vi "RunMeas.vi"(8 "error in (no error)":errorcluster, 11 "NhRegenGridSim in":refnum<class "NHRGridSim.lvclass">) -> (0 "error out":errorcluster, 2 "variant":variant, 3 "NhRegenGridSim out":refnum<class "NHRGridSim.lvclass">)   [LabVIEW 2018, in "AcPwrPlugins.lvlib" / "NHRGridSim.lvclass"]
doc: "This VI acquires data from the instrument and fetches the data from instrument memory into LabVIEW memory."
uses:
  NHRGridSim.lvclass
  AcPwrShared/clMeasurmentData.ctl
  AcPwrShared/clAcPwrAttributes.ctl
  <instrlib>/NH Research 9400 Series/Public/Data/Read Waveform (Current).vi
  <instrlib>/NH Research 9400 Series/Public/Data/Read Waveform (Voltage).vi
  <instrlib>/NH Research 9400 Series/NH Research 9400 Series.lvlib
  AcPwrShared/AcPwrShared.lvlib
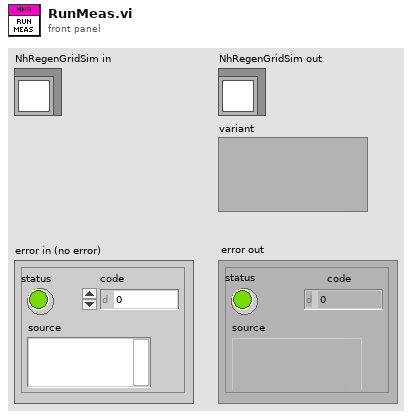
[diagram p1: front panel]
types:
  T1 = typedef "AcPwrPlugins.lvlib/NHRGridSim.lvclass/Device(s)Settings.ctl" = cluster{"MeasName":string, "Modules":T2}
  T2 = typedef "AcPwrPlugins.lvlib/NHRGridSim.lvclass/Modules.ctl" = cluster{"Measurement":cluster{"ApertureLength (s)":dbl, "NumberOfSamples":u32}, "Ranges":cluster{"Irange (A)":dbl, "Vrange (V)":dbl}, "Mode":u8, "Handle":string, "FreqOut (Hz)":dbl, "Connected":bool, "btnIdQuery":bool, "btnReset":bool, "Initialize Timeout ( ms)":u32, "Phase (0: All)":i32, "WatchDog":cluster{"Enable WatchDog":bool, "Robust WatchDog":bool, "Watchdog Interval (s)":dbl}, "Safety Limits":cluster{"Min Voltage (V)":dbl, "Min Voltage Time (s)":dbl, "Max Voltage (V)":dbl, "MaxVoltage Time (s)":dbl, "Max Source Amps (A)":dbl, "Max Source Amps Time (s)":dbl, "Max Sink Amps (A)":dbl, "Max Sink Amps Time (s)":dbl, "Max Source Power (W)":dbl, "Max Source Power Time (s)":dbl, "Max Sink Power (W)":dbl, "Max Sink Power Time (s)":dbl, "Peak Voltage (V)":dbl, "Peak Voltage Enable":bool, "Peak Amps (A)":dbl, "Peak Amps Enable":bool}, "Phases":cluster{"Pout (W)":dbl, "Iout (A)":dbl, "PhaseAngle":dbl, "Vout (V)":dbl, "Phase Name":string}[], "Regulation Gain":dbl, "ChangeOntheFly":bool, "Synchronize Output \nto Phase":bool, "Slew Rate":cluster{"Voltage Slew (Volts/s)":dbl, "Phase Angle (Degrees/s)":dbl}}[]
  T3 = typedef "AcPwrPlugins.lvlib/NHRGridSim.lvclass/Measurements.ctl" = cluster{"Handle":string, "Name":string, "Enabled ":bool, "Measurement Value":dbl, "Phase ":i32, "Measurement Type ":T4}[]
  T4 = typedef "AcPwrPlugins.lvlib/NHRGridSim.lvclass/MeasurementType.ctl" = enum16{"Average Current", "Average Voltage"}
  T5 = typedef "AcPwrShared.lvlib/clMeasurmentData.ctl" = cluster{"MeasName":string, "XML Data":string, "WaveformData":waveform(dbl)[]}
  T6 = typedef "AcPwrShared.lvlib/clAcPwrAttributes.ctl" = cluster{"ProtectionStatusString":string, "Handle_MeasurementType":string, "Status Byte Register":cluster{"Busy":bool, "Remote Mode":bool, "Error in Queue":bool, "QUES=Questionable Status Summary":bool, "MAV = Message Available":bool, "ESB = Event Status Byte Summary":bool, "RQS = Request for Service":bool, "OPER = Operation Event Summary":bool}}
  T7 = cluster{"Busy":bool, "Remote Mode":bool, "Error in Queue":bool, "QUES = Questionable Status Summary":bool, "MAV = Message Available":bool, "ESB = Event Status Byte Summary":bool, "RQS = Request for Service":bool, "OPER = Operation Event Summary":bool}
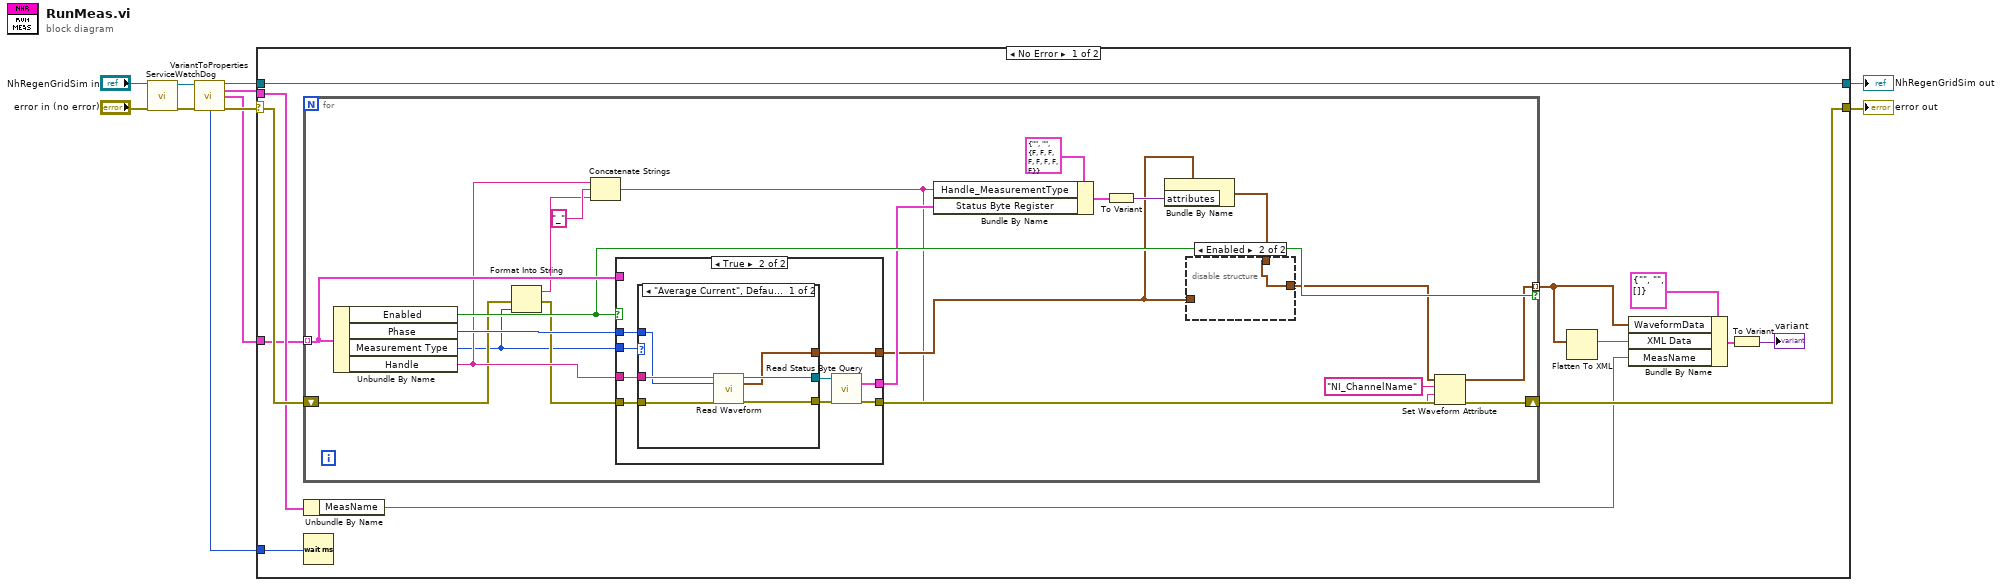
[diagram p0: block diagram]
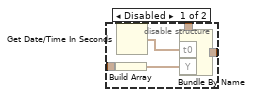
[diagram p2: hidden frame]
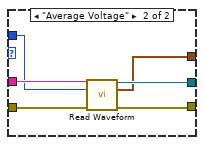
[diagram p4: hidden frame]
diagram:
  n1 = call-dynamic "ServiceWatchDog.vi"("error in (no error)"="error in (no error)", "NHRGridSim in"="NhRegenGridSim in") -> ("error out"=w4:errorcluster, "NHRGridSim out"=w3:refnum<class "NHRGridSim.lvclass">)  [unwired: 8 in]
  n2 = call "VariantToProperties.vi"("NHRGridSim in"=w3, "error in (no error)"=w4) -> ("NHRGridSim out"=w9:refnum<class "NHRGridSim.lvclass">, "Device(s)Settings"=w7:T1, "Measurements"=w5:T3, "Measurement Refresh Time (ms)"=w6:u32, "error out"=w8:errorcluster)  [unwired: 7 in, 2 out]
  n3 = case shown="No Error" w8 {
    selector: w8 -> [w22 w73]
    tunnel: [w21 w73] -> w11
    tunnel: [w23 w74] -> w10
    tunnel: w9 -> [w23 w74]
    tunnel: w7 -> [w20 _]
    tunnel: w6 -> [w19 _]
    tunnel: w5 -> [w18 _]
    frame No Error {
      n4 = for {
        tunnel: w18 -> [w44] mode=indexing
        shift-right: [w28] -> w21
        shift-left: w22 -> [w37]
        tunnel: [w26] -> w12 mode=indexing if=w42
        n5 = Unbundle By Name(w44) -> ("Enabled"=w42:bool, "Phase"=w43:i32, "Measurement Type"=w35:T4, "Handle"=w38:string)
        n6 = Format Into String(error in=w37, w35) -> (resulting string=w34:string, error out=w36:errorcluster)  [unwired: 2 in]
        n7 = Concatenate Strings(w38, "_", w34) -> (w24:string)
        n8 = case shown="True" w42 {
          tunnel: w44 -> [_ _]
          tunnel: w36 -> [w51 w58]
          tunnel: w38 -> [_ w57]
          tunnel: [w51 w56] -> w27
          tunnel: w43 -> [_ w59]
          tunnel: w35 -> [_ w60]
          tunnel: [_ w55] -> w30
          tunnel: [_ w54] -> w32
          frame False {
          }
          frame True {
            n9 = case shown="\"Average Current\", Default" w60 {
              tunnel: w59 -> [w63 w68]
              tunnel: w58 -> [w66 w71]
              tunnel: w57 -> [w64 w70]
              tunnel: [w65 w72] -> w52
              tunnel: [w62 w69] -> w53
              tunnel: [w61 w67] -> w55
              frame "Average Current", Default {
                n10 = call-poly <instrlib>:"Read Waveform.vi"("VISA resource name"=w64, "Phase (0: All)"=w63, "error in (no error)"=w66) -> ("VISA resource name out"=w62:refnum<visa-resource-name>, "Waveform (A)"=w61:waveform(dbl), "error out"=w65:errorcluster)  [unwired: 10 in]
              }
              frame "Average Voltage" {
                n11 = call-poly <instrlib>:"Read Waveform.vi"("VISA resource name"=w70, "Phase (0: All)"=w68, "error in (no error)"=w71) -> ("VISA resource name out"=w69:refnum<visa-resource-name>, "Waveform (V)"=w67:waveform(dbl), "error out"=w72:errorcluster)  [unwired: 10 in]
              }
            }
            n12 = call <instrlib>:"Read Status Byte Query.vi"("VISA resource name"=w53, "error in (no error)"=w52) -> ("Status Byte Register"=w54:T7, "error out"=w56:errorcluster)  [unwired: 11 in, 1 out]
          }
        }
        n13 = Bundle By Name(cluster=T6 {"ProtectionStatusString"="", "Handle_MeasurementType"="", "Status Byte Register"={"Busy"=FALSE, "Remote Mode"=FALSE, "Error in Queue"=FALSE, "QUES=Questionable Status Summary"=FALSE, "MAV = Message Available"=FALSE, "ESB = Event Status Byte Summary"=FALSE, "RQS = Request for Service"=FALSE, "OPER = Operation Event Summary"=FALSE}} ("Attributes"), "Handle_MeasurementType"=w24, "Status Byte Register"=w32) -> (w31:T6)
        n14 = To Variant(anything=w31) -> (Variant=w41:variant)
        n15 = Bundle By Name(cluster=w30, "attributes"=w41) -> (w39:waveform(dbl))
        n16 = disable-structure shown="Enabled" {
          disable-tunnel: [w47 w50] -> w25
          disable-tunnel: w39 -> [w46 w50]
          disable-tunnel: w30 -> [w45 _]
          frame Disabled {
            n17 = Build Array(w45) -> (w49:waveform(dbl)[])
            n18 = Get Date/Time In Seconds() -> (seconds since 1Jan1904=w48:timestamp)
            n19 = Bundle By Name(cluster=w46, "t0"=w48, "Y"=w49) -> (w47:waveform(dbl))
          }
          frame Enabled {
          }
        }
        n20 = Set Waveform Attribute(4:w27, 5:w24, 6:"NI_ChannelName" ("name"), 7:w25) -> (0:w28:errorcluster, 3:w26:waveform(dbl))  [unwired: 1 out]
      }
      n21 = Unbundle By Name(w20) -> ("MeasName"=w13:string)
      n22 = Wait (ms)(milliseconds to wait=w19) -> ()  [unwired: 1 out]
      n23 = Flatten To XML(anything=w12) -> (xml string=w15:string)
      n24 = Bundle By Name(cluster=T5 {"MeasName"="", "XML Data"="", "WaveformData"=[]} ("MeasurmentDataCluster"), "WaveformData"=w12, "XML Data"=w15, "MeasName"=w13) -> (w16:T5)
      n25 = To Variant(anything=w16) -> (Variant=→"variant":variant)
    }
    frame Error {
    }
  }
  "NhRegenGridSim out" <- w10
  "error out" <- w11
